vi "1_OnInterrupts_Raw_Slow.vi"() -> ()   [LabVIEW 2020]
uses:
  <vilib>/Instr/_visa.llb/VISA Configure Serial Port (Instr).vi
  <vilib>/Analysis/NI_AALBase.lvlib
panel:
  in  "stop":bool
  in  "Tab Control":enum32{"Main", "Service"}(tab)
  out "mean":dbl=672.206 format="%.6f"
  out "standard deviation":dbl=7.149110683653894 format="%.6f"
  out "Measurement":u8[](graph)
  out "error out":errorcluster
  in  "VISA resource name":refnum<visa-resource-name>="COM7"
  out "answer":string="673 \n\r"
  in  "Clear":bool
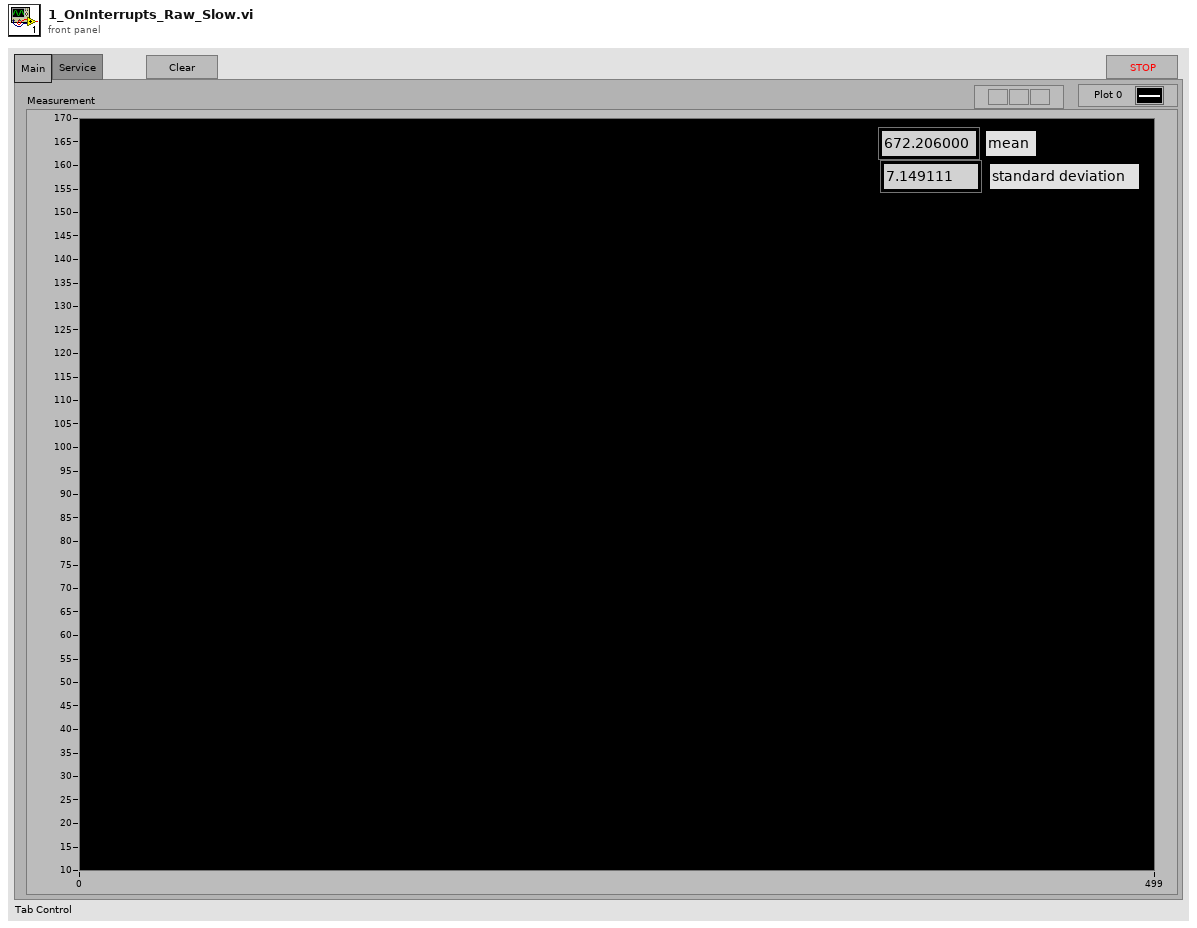
[diagram p1: front panel]
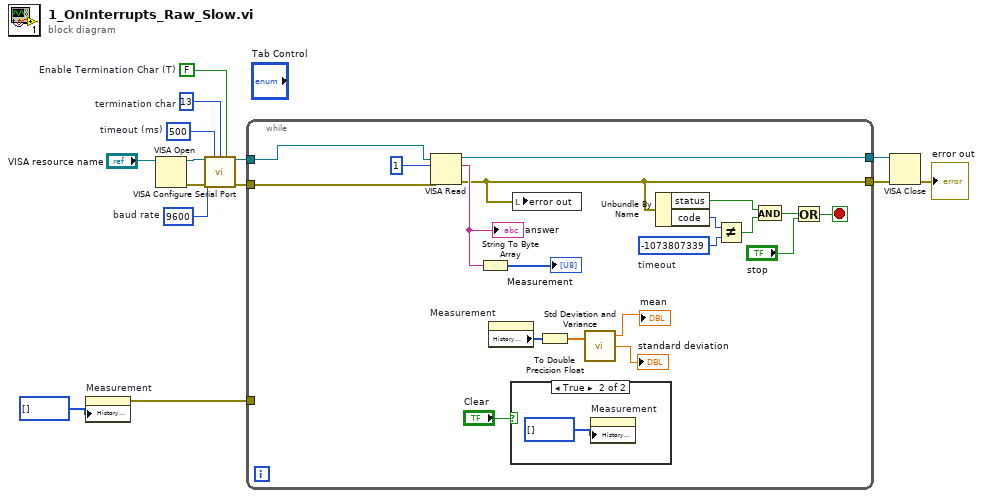
[diagram p0: block diagram]
diagram:
  w3 = u32 9600  # baud rate
  w4 = u32 500  # timeout (ms)
  w10 = FALSE  # Enable Termination Char (T)
  w11 = u8 13  # termination char
  n1 = property on="Measurement" class="WFChart (strict)"("History Data"=u8[] []) -> (error out=w1:errorcluster)  [unwired: 2 in, 1 out]
  n2 = VISA Open(VISA resource name="VISA resource name") -> (VISA resource name=w13:refnum<visa-resource-name>, error out=w14:errorcluster)  [unwired: 4 in]
  n3 = call-poly "VISA Configure Serial Port"("VISA resource name"=w13, "timeout (10sec)"=w4, "termination char\n(0xA = '\\n' = LF)"=w11, "Enable Termination\nChar (T)"=w10, "baud rate (9600)"=w3, "error in (no error)"=w14) -> ("VISA resource name out"=w7:refnum<visa-resource-name>, "error out"=w6:errorcluster)  [unwired: 8 in]
  n4 = while {
    tunnel: w7 -> [w32]
    tunnel: [w33] -> w9
    tunnel: w6 -> [w16]
    tunnel: [w25] -> w8
    tunnel: w1 -> [_]
    stop <- w19 stop-if-true
    w23 = -1073807339  # timeout
    n5 = VISA Read(VISA resource name=w32, byte count=u32 1, error in (no error)=w16) -> (VISA resource name out=w33:refnum<visa-resource-name>, read buffer=w30:string, error out=w25:errorcluster)  [unwired: 1 out]
    "answer" <- w30
    n6 = String To Byte Array(string=w30) -> (unsigned byte array=→"Measurement":u8[])
    n7 = property on="Measurement" class="WFChart (strict)"() -> ("History Data"=w29:u8[])  [unwired: 2 in, 2 out]
    n8 = case shown="True" "Clear" {
      frame False {
      }
      frame True {
        n9 = property on="Measurement" class="WFChart (strict)"("History Data"=u8[] []) -> ()  [unwired: 2 in, 2 out]
      }
    }
    n10 = local write "error out"(w25) -> ()
    n11 = To Double Precision Float(number=w29) -> (double precision float=w15:dbl[])
    n12 = call <vilib>:"Std Deviation and Variance.vi"("X"=w15) -> ("mean"=→"mean":dbl, "standard deviation"=→"standard deviation":dbl)  [unwired: 1 in, 1 out]
    n13 = Unbundle By Name(w25) -> ("status"=w21:bool, "code"=w24:i32)
    n14 = Not Equal?(x=w24, y=w23) -> (x != y?=w22:bool)
    n15 = And(x=w21, y=w22) -> (x .and. y?=w20:bool)
    n16 = Or(x=w20, y="stop") -> (x .or. y?=w19:bool)
  }
  n17 = VISA Close(VISA resource name=w9, error in (no error)=w8) -> (error out=→"error out":errorcluster)
